vi "test Loopback RT to BC with Start and Stop.vi"(8 "error in":errorcluster, 11 "TestCase in":refnum<class "Loopback.lvclass">) -> (0 "error out":errorcluster, 3 "TestCase out":refnum<class "Loopback.lvclass">)   [LabVIEW 2020, in "Loopback.lvclass"]
uses:
  Loopback.lvclass
  C:/dev/niveristand-custom-device-testing-tools/VeriStandTestCase/VeriStandTestCase.lvclass
  <vilib>/numeric/Random Number (Range) U64.vi
  485b7c2b-8320-4722-9ec7-d01f27c65546.vi
  1571aa8d-489e-4c94-925a-256c0ab49a50.vi
  a09b07c8-52ad-4e58-9957-78b331af32de.vi
  9426a44b-b3d4-42e7-bade-e6518c4f8208.vi
  <vilib>/numeric/sub_Random U32.vi
  <vilib>/NI VeriStand/Execution/Workspace/NI VeriStand - Set Multiple Channel Values.vi
  <vilib>/NI VeriStand/Execution/Workspace/NI VeriStand - Get Multiple Channel Values.vi
  <vilib>/NI VeriStand/Execution/Workspace/NI VeriStand - Set Single Channel Value.vi
  <vilib>/addons/_JKI Toolkits/VI Tester/TestCase.llb/TestCase.lvclass
  <vilib>/NI VeriStand/Execution/Workspace/NI_VS Workspace ExecutionAPI.lvlib
  C:/Program Files (x86)/National Instruments/LabVIEW 2020/vi.lib/addons/_JKI Toolkits/VI Tester/TestCase.llb/TestCase.lvclass
  C:/dev/niveristand-ballard-milStd1553-custom-device/Source/Custom Device Support/Tests/System/Loopback/Loopback.lvclass
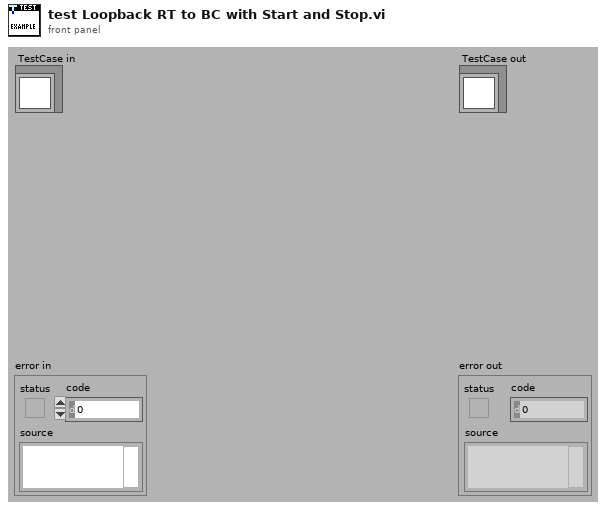
[diagram p1: front panel]
types:
  T1 = typedef "NI_VS Workspace ExecutionAPI.lvlib/WorkspaceAPI.ctl" = refnum<k24>
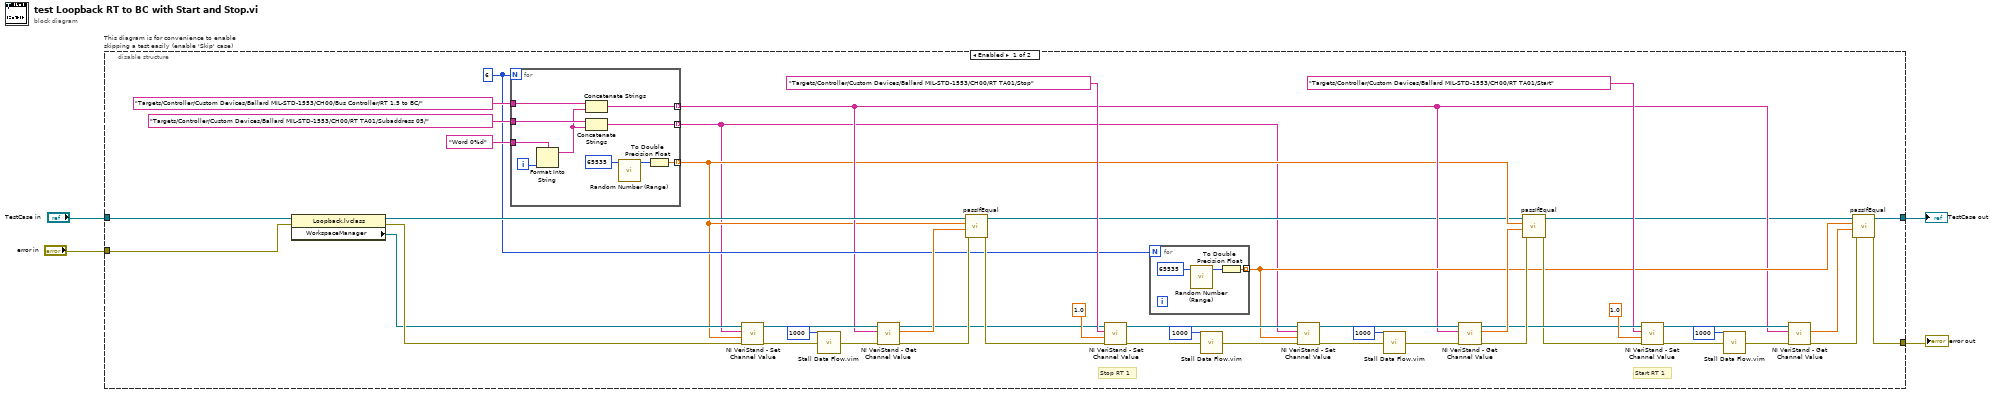
[diagram p0: block diagram]
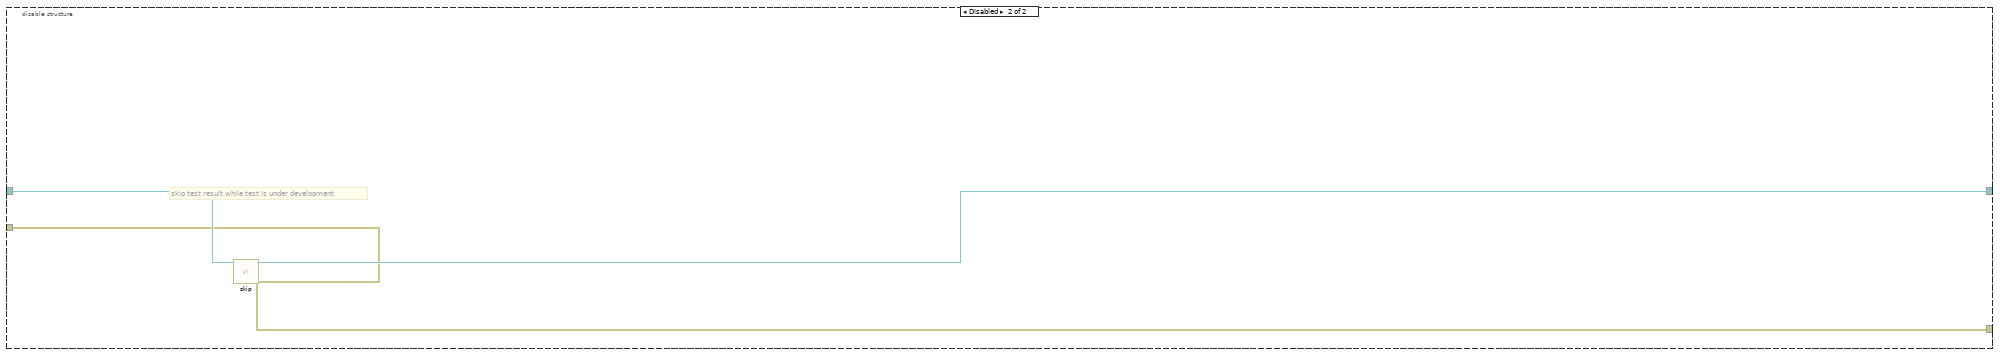
[diagram p2: hidden frame]
diagram:
  n1 = disable-structure "This diagram is for convenience to enable skipping a test easily (enable 'Skip' case)" shown="Enabled" {
    disable-tunnel: "TestCase in" -> [w42 w68]
    disable-tunnel: [w6 w66] -> w1
    disable-tunnel: [w10 w67] -> w3
    disable-tunnel: "error in" -> [w39 w65]
    frame Enabled {
      w13 = 6
      # "Start RT 1"
      # "Stop RT 1"
      n2 = property class="Loopback.lvclass"(reference=w42, error in=w39) -> (reference out=w51:refnum<class "Loopback.lvclass">, error out=w46:errorcluster, "WorkspaceManager"=w44:T1)
      n3 = for {
        N: w13 -> [_]
        tunnel: "Targets/Controller/Custom Devices/Ballard MIL-STD-1553/CH00/RT TA01/Subaddress 05/" ("Channel") -> [w63]
        tunnel: [w64] -> w5 mode=indexing
        tunnel: "Targets/Controller/Custom Devices/Ballard MIL-STD-1553/CH00/Bus Controller/RT 1.5 to BC/" ("Channel") -> [w62]
        tunnel: [w61] -> w12 mode=indexing
        tunnel: "Word 0%d" -> [w59]
        tunnel: [w55] -> w11 mode=indexing
        i -> [w60]
        n4 = Format Into String(format string=w59, w60) -> (resulting string=w58:string)  [unwired: 2 in, 1 out]
        n5 = Concatenate Strings(w62, w58) -> (w61:string)
        n6 = Concatenate Strings(w63, w58) -> (w64:string)
        n7 = call-poly <vilib>:"Random Number (Range).vi"("upper bound (100)"=u64 65535) -> ("number"=w57:u64)  [unwired: 10 in]
        n8 = To Double Precision Float(number=w57) -> (double precision float=w55:dbl)
      }
      n9 = call-poly <vilib>:"NI VeriStand - Set Channel Value.vi"("error in (no error)"=w46, "Values"=w11, "Channels"=w5, "WorkspaceManager in"=w44) -> ("error out"=w48:errorcluster, "WorkspaceManager out"=w50:T1)  [unwired: 6 in]
      n10 = call "Stall Data Flow.vim"("value in"=w48, "milliseconds to wait"=u32 1000) -> ("value out"=w49:errorcluster)  [unwired: 1 out]
      n11 = call-poly <vilib>:"NI VeriStand - Get Channel Value.vi"("error in (no error)"=w49, "Channels"=w12, "WorkspaceManager in"=w50) -> ("error out"=w45:errorcluster, "Values"=w43:dbl[], "WorkspaceManager out"=w9:T1)  [unwired: 6 in]
      n12 = call-dynamic "passIfEqual.vi"("error in (no error)"=w45, "y"=w43, "x"=w11, "TestCase in"=w51) -> ("error out"=w14:errorcluster, "TestCase out"=w8:refnum<class "Loopback.lvclass">)  [unwired: 6 in]
      n13 = call-poly <vilib>:"NI VeriStand - Set Channel Value.vi"("error in (no error)"=w14, "Value"=1.0, "Channel"="Targets/Controller/Custom Devices/Ballard MIL-STD-1553/CH00/RT TA01/Stop", "WorkspaceManager in"=w9) -> ("error out"=w16:errorcluster, "WorkspaceManager out"=w35:T1)  [unwired: 6 in]
      n14 = for {
        N: w13 -> [_]
        tunnel: [w52] -> w21 mode=indexing
        n15 = call-poly <vilib>:"Random Number (Range).vi"("upper bound (100)"=u64 65535) -> ("number"=w53:u64)  [unwired: 10 in]
        n16 = To Double Precision Float(number=w53) -> (double precision float=w52:dbl)
      }
      n17 = call "Stall Data Flow.vim"("value in"=w16, "milliseconds to wait"=u32 1000) -> ("value out"=w15:errorcluster)  [unwired: 1 out]
      n18 = call-poly <vilib>:"NI VeriStand - Set Channel Value.vi"("error in (no error)"=w15, "Values"=w21, "Channels"=w5, "WorkspaceManager in"=w35) -> ("error out"=w19:errorcluster, "WorkspaceManager out"=w34:T1)  [unwired: 6 in]
      n19 = call "Stall Data Flow.vim"("value in"=w19, "milliseconds to wait"=u32 1000) -> ("value out"=w18:errorcluster)  [unwired: 1 out]
      n20 = call-poly <vilib>:"NI VeriStand - Get Channel Value.vi"("error in (no error)"=w18, "Channels"=w12, "WorkspaceManager in"=w34) -> ("error out"=w33:errorcluster, "Values"=w32:dbl[], "WorkspaceManager out"=w30:T1)  [unwired: 6 in]
      n21 = call-dynamic "passIfEqual.vi"("error in (no error)"=w33, "y"=w32, "x"=w11, "TestCase in"=w8) -> ("error out"=w26:errorcluster, "TestCase out"=w7:refnum<class "Loopback.lvclass">)  [unwired: 6 in]
      n22 = call-poly <vilib>:"NI VeriStand - Set Channel Value.vi"("error in (no error)"=w26, "Value"=1.0, "Channel"="Targets/Controller/Custom Devices/Ballard MIL-STD-1553/CH00/RT TA01/Start", "WorkspaceManager in"=w30) -> ("error out"=w27:errorcluster, "WorkspaceManager out"=w22:T1)  [unwired: 6 in]
      n23 = call "Stall Data Flow.vim"("value in"=w27, "milliseconds to wait"=u32 1000) -> ("value out"=w23:errorcluster)  [unwired: 1 out]
      n24 = call-poly <vilib>:"NI VeriStand - Get Channel Value.vi"("error in (no error)"=w23, "Channels"=w12, "WorkspaceManager in"=w22) -> ("error out"=w24:errorcluster, "Values"=w25:dbl[])  [unwired: 6 in, 1 out]
      n25 = call-dynamic "passIfEqual.vi"("error in (no error)"=w24, "y"=w25, "x"=w21, "TestCase in"=w7) -> ("error out"=w10:errorcluster, "TestCase out"=w6:refnum<class "Loopback.lvclass">)  [unwired: 6 in]
    }
    frame Disabled {
      # "skip test result while test is under development"
      n26 = call <vilib>:"skip.vi"("error in (no error)"=w65, "TestCase in"=w68) -> ("error out"=w67:errorcluster, "TestCase out"=w66:refnum<class "Loopback.lvclass">)  [unwired: 8 in]
    }
  }
  "error out" <- w3
  "TestCase out" <- w1
